vi "SOUR_POW_LEV_SLOP.vi"(0 "VISA IN":refnum<visa-resource-name>, 1 "Slope Value(db/GHz)":i32, 5 "error in":errorcluster, 7 "Channel":i32) -> (14 "VISA Out":refnum<visa-resource-name>, 19 "error out":errorcluster)   [LabVIEW 2018, in "PNA-X.lvlib"]
doc: "SOURce<cnum>:POWer[:LEVel]:SLOPe <num> \n(Read-Write) Sets the RF power slope value. \nParameters \n<cnum> Any existing channel number. If unspecified, value is set to 1 \n<num> Slope value in db/GHz. Choose any integer between -2 and 2 (0 is no slope). \nExamples SOUR:POW:SLOP 2 \nsource2:power:slope -2 \nQuery Syntax SOURce<cnum>:POWer[:LEVel]:SLOPe? \nReturn Type Numeric \nDefault 0"
uses:
  PNA-X.lvlib
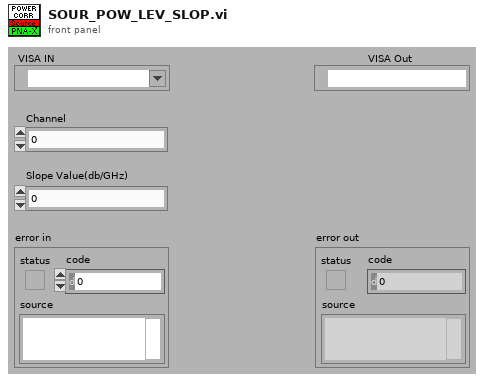
[diagram p1: front panel]
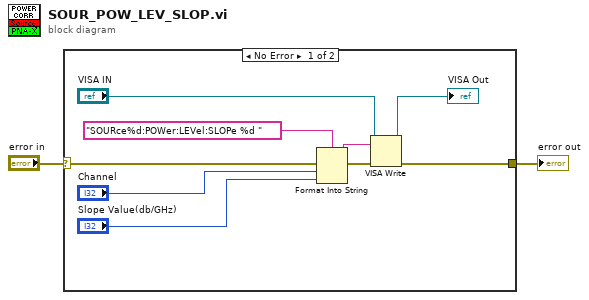
[diagram p0: block diagram]
diagram:
  n1 = case shown="No Error" "error in" {
    selector: "error in" -> [w11 w12]
    tunnel: [w6 w12] -> w1
    frame No Error {
      n2 = Format Into String(format string="SOURce%d:POWer:LEVel:SLOPe %d " ("Cmdline"), error in=w11, "Channel", "Slope Value(db/GHz)") -> (resulting string=w9:string, error out=w10:errorcluster)  [unwired: 1 in]
      n3 = VISA Write(VISA resource name="VISA IN", write buffer=w9, error in (no error)=w10) -> (VISA resource name out=→"VISA Out":refnum<visa-resource-name>, error out=w6:errorcluster)  [unwired: 1 out]
    }
    frame Error {
    }
  }
  "error out" <- w1
